vi "Lezeti_Power_Monitor_16_b.vi"() -> ()   [LabVIEW 2015]
doc: "This example shows how to use autosetup and acquire a waveform on a single channel."
uses:
  LEZETI/LabView/Lezeti_Power_Monitor_03/Public/Data/Read (Multiple Waveforms).vi
  <vilib>/measure/madcrms.llb/Basic Averaged DC-RMS for 1 Chan.vi
  <vilib>/addons/Electrical Power/Basic/Measurement/Power (1 Channel).vi
  <vilib>/measure/mascope.llb/Cycle Average and RMS 1 chan.vi
  <vilib>/Utility/file.llb/Write To Spreadsheet File (DBL).vi
  LEZETI/LabView/Lezeti_Power_Monitor_03/RIGOL DS1000 Series.lvlib
  <vilib>/measure/NI_MAPro.lvlib
  <vilib>/addons/Electrical Power/Basic/NI_EP_Basic.lvlib
panel:
  out "Apparent Power (VA)":dbl(graph)
  out "Power Factor":dbl(graph)
  out "Power (Watts)":dbl(graph)
  out "Reactive Power (VAR)":dbl(graph)
  out "Power Factor":dbl
  out "Apparent Power (VA)":dbl
  out "Run Date":string
  out "Run Time":string
  out "Elapsed Time (s)":dbl
  in  "Output File":path
  out "Average Power (Watts)":dbl
  out "Instant Power Waveform":waveform(dbl)(graph)
  out "IRMS":dbl
  out "Current Waveform":waveform(dbl)(graph)
  out "VRMS":dbl
  in  "Stop":bool
  out "Voltage Waveform":waveform(dbl)(graph)
  in  "VISA resource name":refnum<visa-resource-name>
  # "For Lezeti Air Conditioning System (Greenpath Tech)\nBy Matsu Thornton\nJuly 2016"
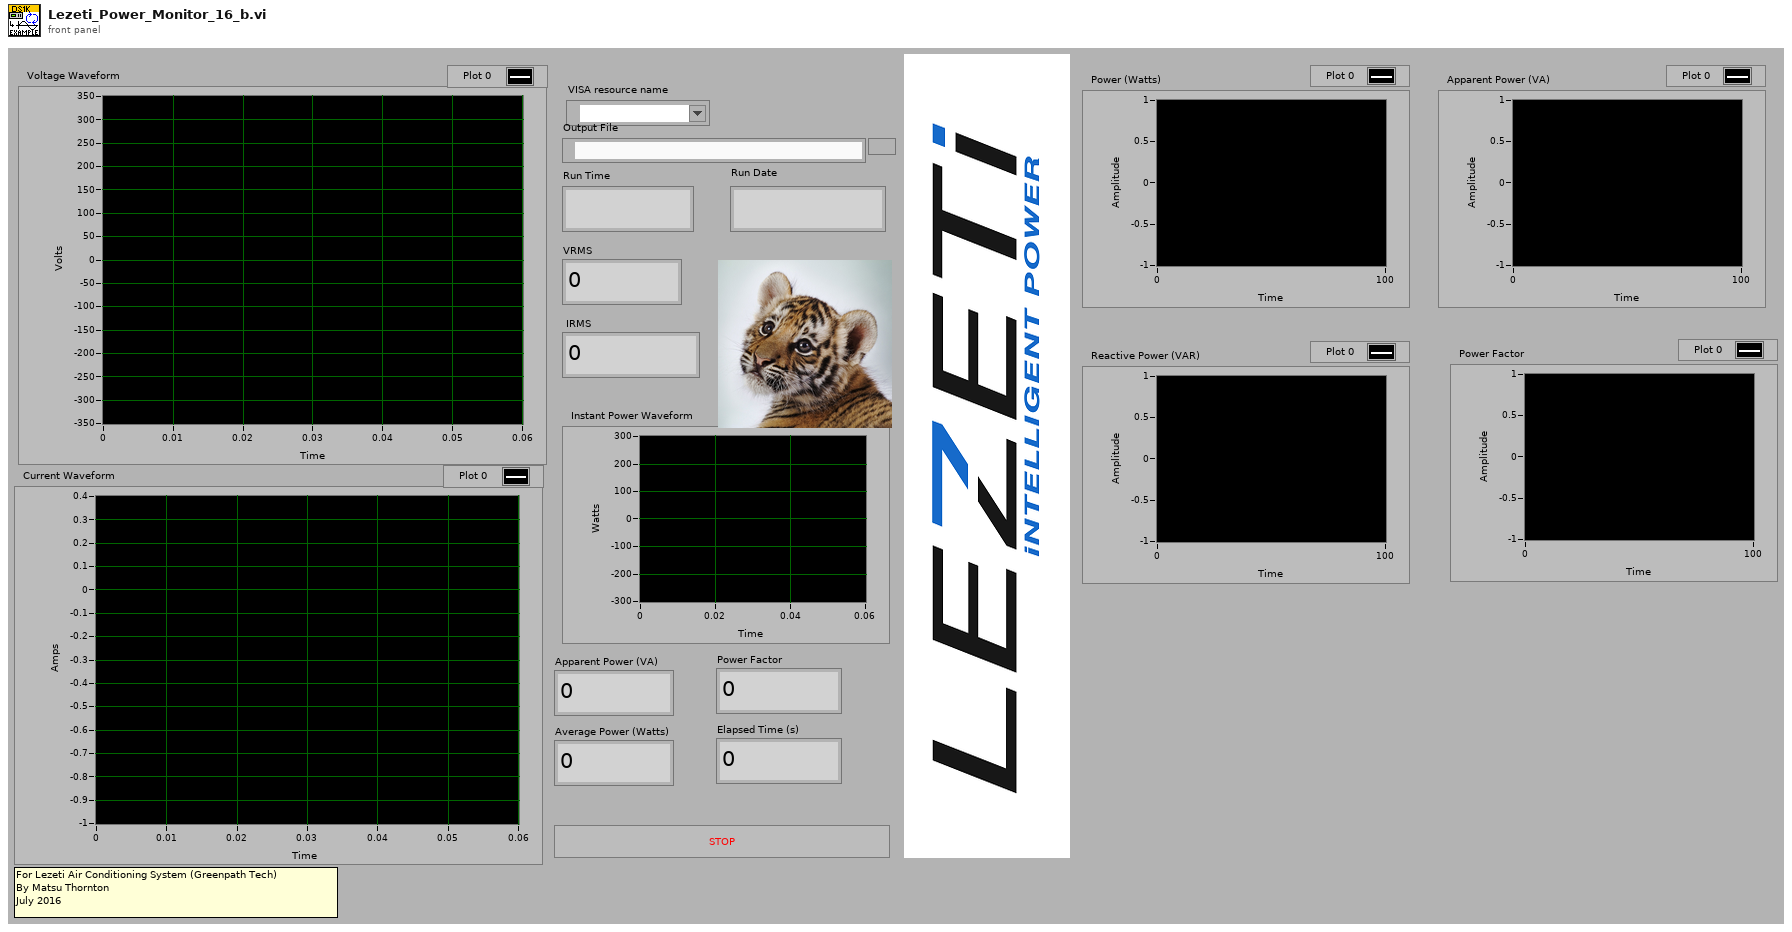
[diagram p1: front panel]
types:
  T1 = typedef "NI_Matrix.lvlib/RealMatrix.ctl" = dbl[][]
  T2 = typedef "NI_EP_Basic.lvlib/basic_Power Value.ctl" = cluster{"active power [W]":dbl, "apparent power [VA]":dbl, "reactive power [VAR]":dbl, "power factor":dbl}
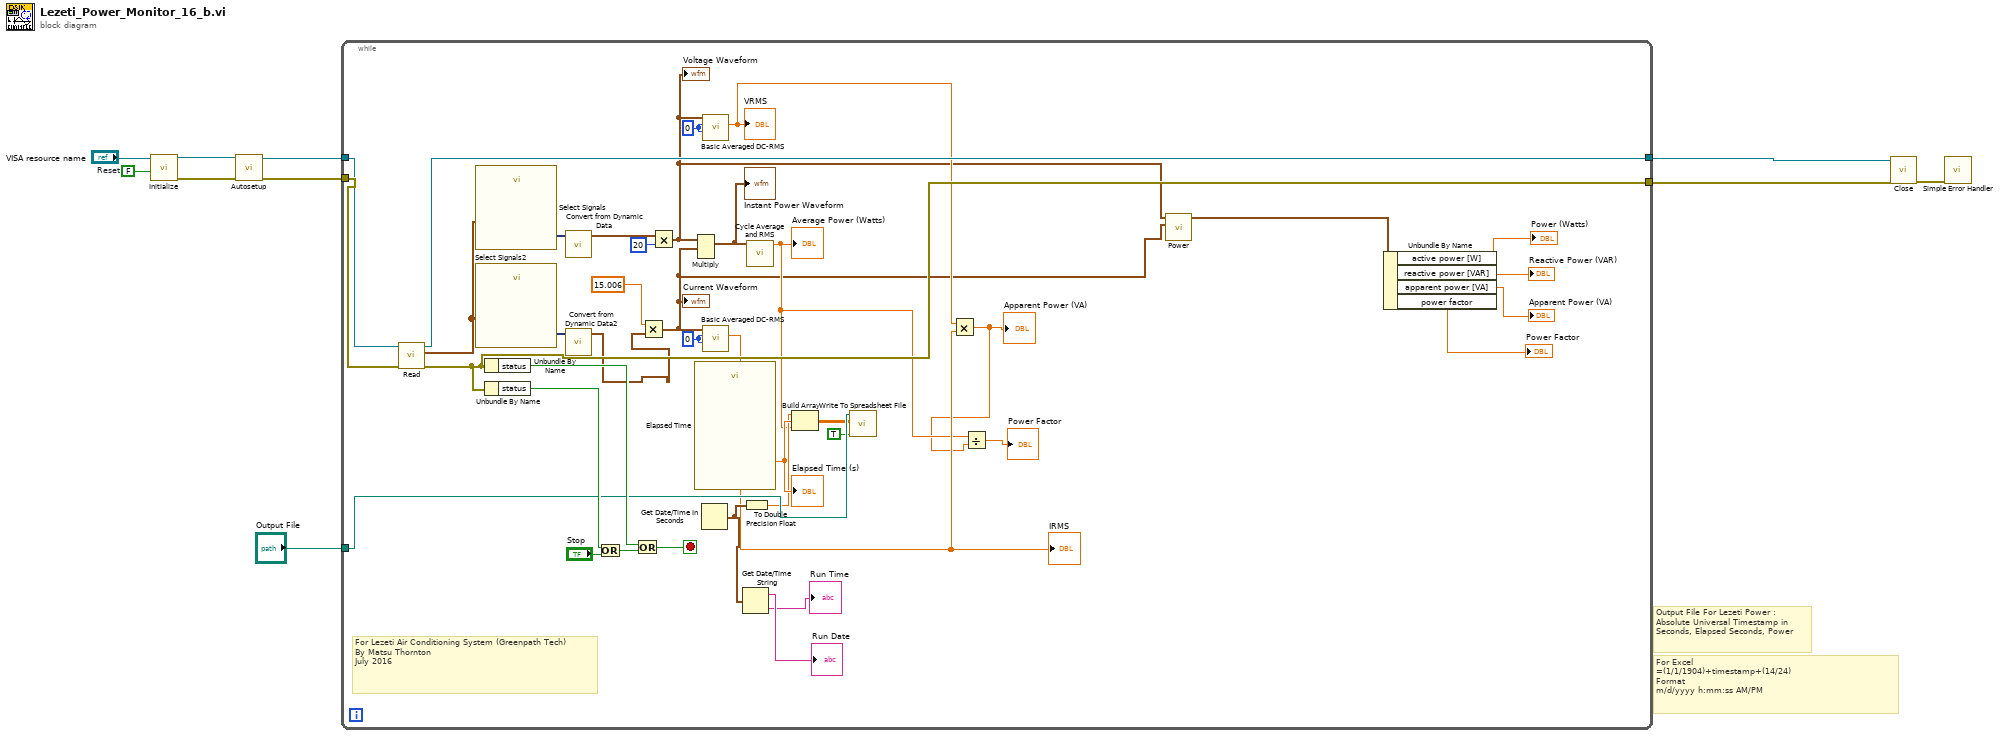
[diagram p0: block diagram]
diagram:
  w3 = FALSE  # Reset
  # "For Excel\n=(1/1/1904)+timestamp+(14/24)\nFormat\nm/d/yyyy h:mm:ss AM/PM"
  # "Output File For Lezeti Power :\nAbsolute Universal Timestamp in Seconds, Elapsed Seconds, Power"
  n1 = call "Initialize.vi"("Reset (True)"=w3, "VISA resource name"="VISA resource name") -> ("error out"=w7:errorcluster, "VISA resource name out"=w6:refnum<visa-resource-name>)  [unwired: 2 in, 6 out]
  n2 = call "Autosetup.vi"("error in (no error)"=w7, "VISA resource name"=w6) -> ("error out"=w4:errorcluster, "VISA resource name out"=w5:refnum<visa-resource-name>)  [unwired: 8 out]
  n3 = while {
    tunnel: w5 -> [w31]
    tunnel: w4 -> [w49]
    tunnel: [w48] -> w9
    tunnel: [w32] -> w2
    tunnel: "Output File" -> [w37]
    stop <- w39 stop-if-true
    w43 = 0
    w45 = 0
    # "For Lezeti Air Conditioning System (Greenpath Tech)\nBy Matsu Thornton\nJuly 2016"
    n4 = call-poly "Read.vi"("error in (no error)"=w49, "VISA resource name"=w31) -> ("error out"=w32:errorcluster, "Waveform Data"=w27:waveform(dbl)[], "VISA resource name out"=w48:refnum<visa-resource-name>)  [unwired: 2 in, 5 out]
    n5 = call "Select Signals"("Signals"=w27) -> ("Signal Out"=w30:dynamicdata)  [unwired: 9 in, 1 out]
    n6 = call "Select Signals2"("Signals"=w27) -> ("Signal Out"=w28:dynamicdata)  [unwired: 9 in, 1 out]
    n7 = Unbundle By Name(w32) -> ("status"=w44:bool)
    n8 = Unbundle By Name(w32) -> ("status"=w47:bool)
    n9 = call "Convert from Dynamic Data"("Dynamic Data Type"=w30) -> ("Waveform"=w29:waveform(dbl))  [unwired: 3 in]
    n10 = call "Convert from Dynamic Data2"("Dynamic Data Type"=w28) -> ("Waveform"=w26:waveform(dbl))  [unwired: 3 in]
    n11 = Or(x=w47, y="Stop") -> (x .or. y?=w40:bool)
    n12 = Or(x=w44, y=w40) -> (x .or. y?=w39:bool)
    n13 = Multiply(x=15.006, y=w26) -> (x*y=w16:waveform(dbl))
    "Current Waveform" <- w16
    n14 = Multiply(x=w29, y=20) -> (x*y=w17:waveform(dbl))
    "Voltage Waveform" <- w17
    n15 = Multiply(1:w16, 2:w17) -> (0:w38:waveform(dbl))  [unwired: 1 in, 1 out]
    "Instant Power Waveform" <- w38
    n16 = call "Elapsed Time"() -> ("Elapsed Time (s)"=w34:dbl)  [unwired: 12 in, 7 out]
    "Elapsed Time (s)" <- w34
    n17 = Get Date/Time In Seconds() -> (seconds since 1Jan1904=w25:timestamp)
    n18 = call-poly <vilib>:"Basic Averaged DC-RMS.vi"("window"=w45, "averaging type"=w45, "signal in"=w17) -> ("RMS value"=w21:dbl)  [unwired: 5 in, 3 out]
    "VRMS" <- w21
    n19 = call-poly <vilib>:"Basic Averaged DC-RMS.vi"("window"=w43, "averaging type"=w43, "signal in"=w16) -> ("RMS value"=w20:dbl)  [unwired: 5 in, 3 out]
    "IRMS" <- w20
    n20 = Get Date/Time String(seconds (now)=w25) -> (date string=→"Run Date":string, time string=→"Run Time":string)  [unwired: 2 in]
    n21 = To Double Precision Float(number=w25) -> (double precision float=w33:dbl)
    n22 = call-poly <vilib>:"Cycle Average and RMS.vi"("signal in"=w38) -> ("cycle average"=w19:dbl)  [unwired: 7 in, 3 out]
    "Average Power (Watts)" <- w19
    n23 = Build Array(w33, w34, w19) -> (w35:T1)
    n24 = call-poly <vilib>:"Write To Spreadsheet File.vi"("append to file? (new file:F)"=TRUE, "2D data"=w35, "file path (dialog if empty)"=w37) -> ()  [unwired: 5 in, 1 out]
    n25 = Multiply(x=w21, y=w20) -> (x*y=w18:dbl)
    "Apparent Power (VA)" <- w18
    n26 = Divide(x=w19, y=w18) -> (x/y=→"Power Factor":dbl)
    n27 = call-poly <vilib>:"Power.vi"("current waveform"=w16, "voltage waveform"=w17) -> ("power value"=w13:T2)  [unwired: 8 in, 1 out]
    n28 = Unbundle By Name(w13) -> ("active power [W]"=→"Power (Watts)":dbl, "reactive power [VAR]"=→"Reactive Power (VAR)":dbl, "apparent power [VA]"=→"Apparent Power (VA)":dbl, "power factor"=→"Power Factor":dbl)
  }
  n29 = call "Close.vi"("error in (no error)"=w2, "VISA resource name"=w9) -> ("error out"=w10:errorcluster)  [unwired: 9 out]
  n30 = call <vilib>:"Simple Error Handler.vi"("error in (no error)"=w10) -> ()  [unwired: 1 in, 8 out]
